vi "get source name.vi"(8 "error in":errorcluster, 11 "timing source in":refnum<class "DAQmx Single Point HW Timed.lvclass">) -> (0 "error out":errorcluster, 2 "source name":string, 3 "timing source out":refnum<class "DAQmx Single Point HW Timed.lvclass">)   [LabVIEW 2014, in "DAQmx Single Point HW Timed.lvclass"]
doc: "Returns the name of the timing source to be used as part of the configuration of a timed loop. For example, the 1 ms timer would return the string \"1 kHz\"."
uses:
  DAQmx Single Point HW Timed.lvclass
  <vilib>/NI/Module Timing Source/timing source/TBM timing source.lvclass
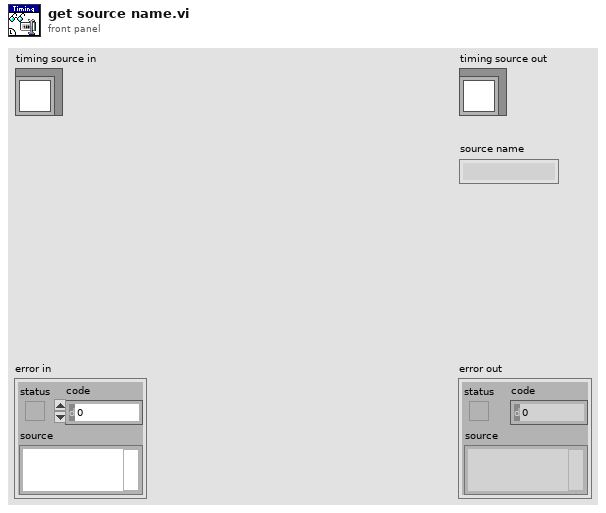
[diagram p1: front panel]
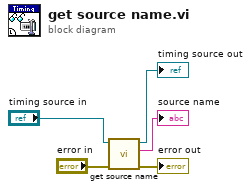
[diagram p0: block diagram]
diagram:
  n1 = call-parent "get source name.vi"("error in"="error in", "timing source in"="timing source in") -> ("error out"=→"error out":errorcluster, "source name"=→"source name":string, "timing source out"=→"timing source out":refnum<class "DAQmx Single Point HW Timed.lvclass">)  [unwired: 7 in]
